vi "ALP2 P.vi"() -> ()   [LabVIEW 2016]
doc: "This VI starts running and asks if it want to adquire data or exit. If the user choose to adquired data the user is allowed to make dynamic changes to the resulting graph so it can best fit the data, also it allows the user to save the data and the folder is already named with the date and time the data was saved. It allows to make a header to the data which is included in the file.\n\nAlexis Lopez\nP350\nCSUSB Physics"
uses:
  typedefs/measurement parameters.ctl
  typedefs/ferro response parameter cluster.ctl
panel:
  in  "date format (0) 2":enum16{"short", "long", "abbreviated"}(ring)
  in  "Stop":bool
  in  "File Header":string="This run was taken on the XXX sample under the following conditions: Temp=..., etc. ...\n\nFormat:\ntime    voltage    fit voltage    fit parameters\n\n<data below>\n\n"
  out "Data to Save":dbl[][](array[numeric])
  in  "Restart":bool
  in  "Save Data":bool
  in  "Fitting Parameters":T1={"amplitude a (V)"=5.0, "time const a (uS)"=15.0, "amplitude b (V)"=10.0, "time const b (uS)"=150.0} {"time const b (uS)" scale=0.0..200.0; "amplitude b (V)" scale=0.0..50.0; "time const a (uS)" scale=0.0..200.0; "amplitude a (V)" scale=0.0..50.0}
  out "Analysis Graph":cluster{"time array (s)":dbl[], dbl[]}[](graph)
  out "Acquisition Graph":T2(graph)
  out "count":i32=100
  in  "Meas Params":T3={"time step (uS)"=1.0, "N meas"=1000, "N meas reps"=100} caption="Measurement Parameters"
  in  "Start":bool
  # "Simulated FerroElectric Experiment"
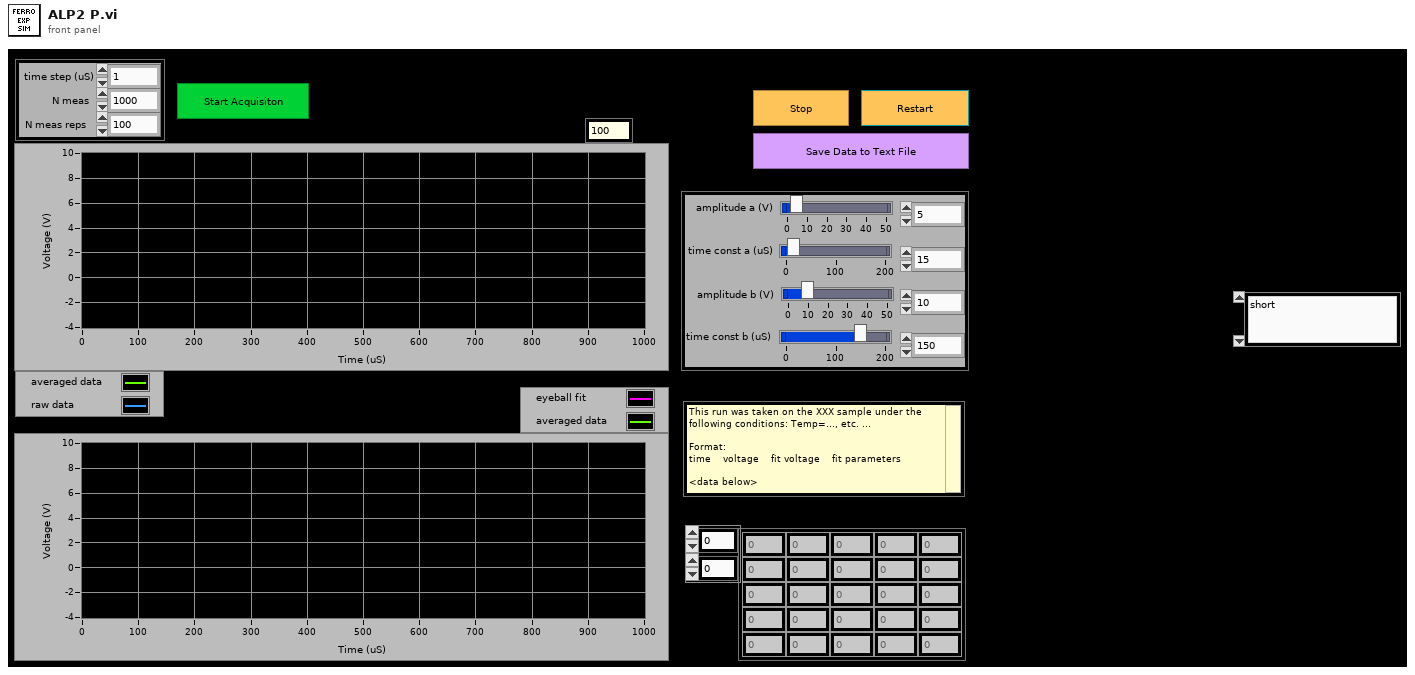
[diagram p1: front panel]
types:
  T1 = typedef "ferro response parameter cluster.ctl" = cluster{"amplitude a (V)":dbl, "time const a (uS)":dbl, "amplitude b (V)":dbl, "time const b (uS)":dbl}
  T2 = cluster{"time array (s)":dbl[], "voltage array (V)":dbl[]}[]
  T3 = typedef "measurement parameters.ctl" = cluster{"time step (uS)":dbl, "N meas":i32, "N meas reps":i32}
  T4 = cluster{"time array (uS)":dbl[], "voltage array (V)":dbl[]}
  T5 = cluster{"time array (uS)":dbl[], "voltage array (V)":dbl[]}[]
  T6 = cluster{"time array out (uS)":dbl[], "voltage array out (V)":dbl[]}
  T7 = cluster{"time array out (uS)":dbl[], "voltage array out (V)":dbl[]}[]
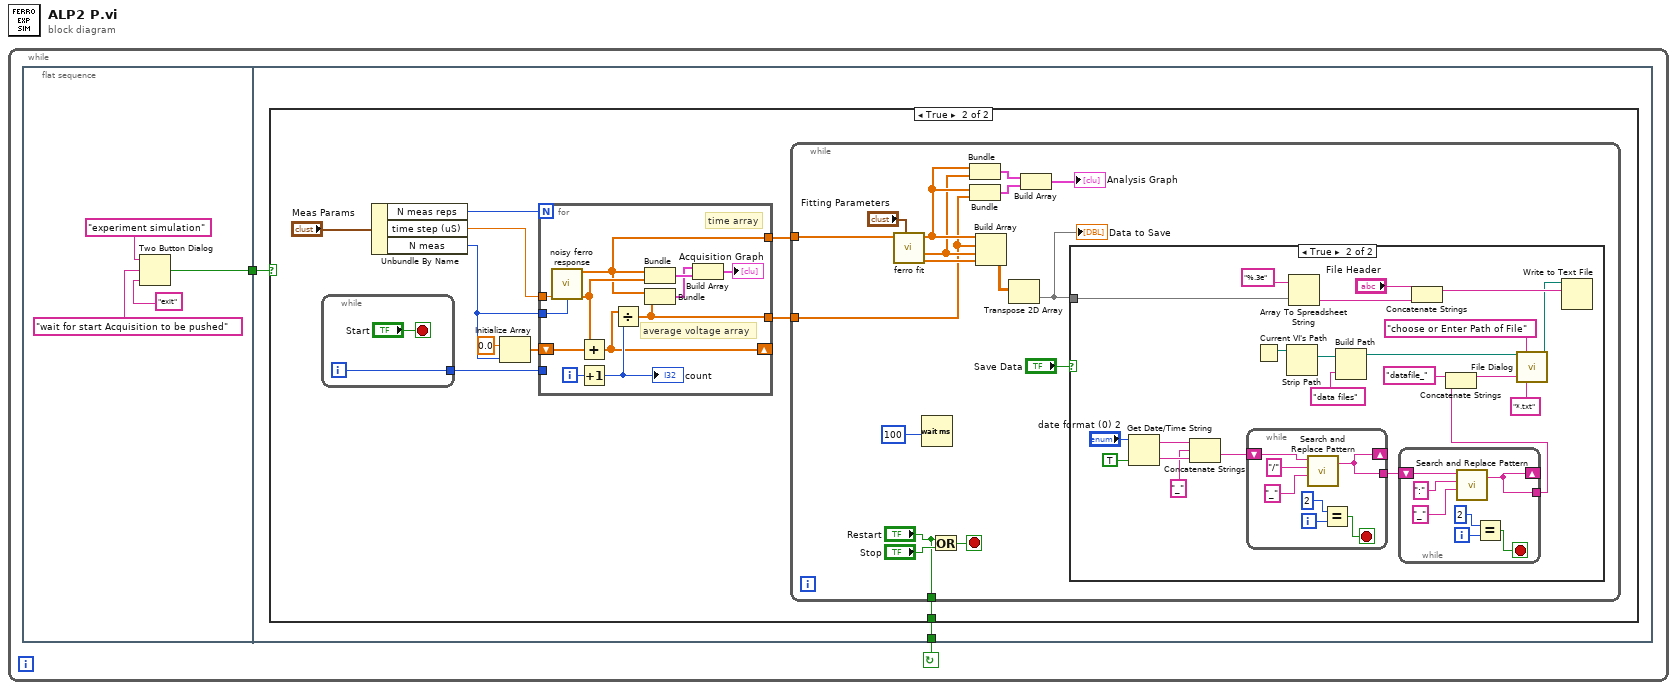
[diagram p0: block diagram]
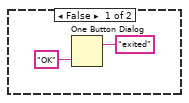
[diagram p2: hidden frame]
diagram:
  n1 = while {
    stop <- w1 continue-if-true
    n2 = flat-sequence {
      tunnel: [w3] -> w2
      tunnel: w2 -> [w8]
      tunnel: [w7] -> w1
      frame #0 {
        n3 = Two Button Dialog(message="experiment simulation", 1:"exit", 2:"wait for start Acquisition to be pushed") -> (T button?=w3:bool)
      }
      frame #1 {
        n4 = case shown="True" w8 {
          tunnel: [_ w11] -> w7
          frame False {
            n5 = One Button Dialog(message="exited", button name ("OK")="OK") -> ()  [unwired: 1 out]
          }
          frame True {
            n6 = while {
              tunnel: [w21] -> w12
              i -> [w21]
              stop <- "Start" stop-if-true
            }
            n7 = Unbundle By Name("Meas Params") -> ("N meas reps"=w15:i32, "time step (uS)"=w19:dbl, "N meas"=w16:i32)
            n8 = Initialize Array(0.0 ("element"), w16) -> (w18:dbl[])
            n9 = for {
              N: w15 -> [_]
              tunnel: w19 -> [w86]
              tunnel: w16 -> [w85]
              shift-right: [w79] -> _
              shift-left: w18 -> [w80]
              tunnel: [w76] -> w14
              tunnel: [w75] -> w13
              tunnel: w12 -> [_]
              i -> [w84]
              # "average voltage array"
              # "time array"
              n10 = call "noisy ferro response.vi"("time step (uS)"=w86, "N meas"=w85) -> ("time array (uS)"=w76:dbl[], "voltage array (V)"=w81:dbl[])  [unwired: 12 in]
              n11 = Add(x=w81, y=w80) -> (x+y=w79:dbl[])
              n12 = Increment(x=w84) -> (x+1=w83:i32)
              "count" <- w83
              n13 = Divide(x=w79, y=w83) -> (x/y=w75:dbl[])
              n14 = Bundle("time array (uS)"=w76, "voltage array (V)"=w81) -> (w78:T4)  [unwired: 1 in]
              n15 = Bundle("time array (uS)"=w76, w75) -> (w77:cluster{"time array (uS)":dbl[], dbl[]})  [unwired: 1 in]
              n16 = Build Array(w77, w78) -> (→"Acquisition Graph":T5)
            }
            n17 = while {
              tunnel: w14 -> [w37]
              tunnel: w13 -> [w28]
              tunnel: ["Restart"] -> w11
              stop <- w24 stop-if-true
              n18 = call "ferro fit.vi"("ferro response parameters"="Fitting Parameters", "time array in (uS)"=w37) -> ("parameters array out"=w31:dbl[], "voltage array out (V)"=w29:dbl[], "time array out (uS)"=w30:dbl[])  [unwired: 7 in]
              n19 = Wait (ms)(milliseconds to wait=u32 100 ("millisecond timer value")) -> ()  [unwired: 1 out]
              n20 = Or(x="Restart", y="Stop") -> (x .or. y?=w24:bool)
              n21 = Bundle("time array out (uS)"=w30, "voltage array out (V)"=w29) -> (w34:T6)  [unwired: 1 in]
              n22 = Bundle("time array out (uS)"=w30, w28) -> (w33:cluster{"time array out (uS)":dbl[], dbl[]})  [unwired: 1 in]
              n23 = Build Array(w30, w28, w29, w31) -> (w35:dbl[][])
              n24 = Transpose 2D Array(2D array=w35) -> (transposed array=w26:dbl[][])
              "Data to Save" <- w26
              n25 = Build Array(w34, w33) -> (→"Analysis Graph":T7)
              n26 = case shown="True" "Save Data" {
                tunnel: w26 -> [_ w60]
                frame False {
                }
                frame True {
                  n27 = Get Date/Time String(date format (0)="date format (0) 2", want seconds? (F)=TRUE) -> (date string=w41:string, time string=w46:string)  [unwired: 1 in]
                  n28 = Concatenate Strings(w41, "_", w46) -> (w44:string)
                  n29 = while {
                    shift-right: [w73] -> _
                    shift-left: w44 -> [w74]
                    tunnel: [w73] -> w45
                    i -> [w72]
                    stop <- w70 stop-if-true
                    n30 = call <vilib>:"Search and Replace Pattern.vi"("string"=w74, "regular expression (\"\")"="/", "replace string (\"\")"="_") -> ("result string"=w73:string)  [unwired: 2 in, 1 out]
                    n31 = Equal?(x=2, y=w72) -> (x = y?=w70:bool)
                  }
                  n32 = Current VI's Path() -> (path=w55:path)
                  n33 = Strip Path(path=w55) -> (stripped path=w49:path)  [unwired: 1 out]
                  n34 = Array To Spreadsheet String(array=w60, 3:"%.3e") -> (spreadsheet string=w57:string)  [unwired: 1 in]
                  n35 = Build Path(base path=w49, name or relative path="data files") -> (appended path=w53:path)
                  n36 = while {
                    shift-right: [w66] -> _
                    shift-left: w45 -> [w67]
                    tunnel: [w66] -> w39
                    i -> [w63]
                    stop <- w64 stop-if-true
                    n37 = call <vilib>:"Search and Replace Pattern.vi"("string"=w67, "regular expression (\"\")"=":", "replace string (\"\")"="_") -> ("result string"=w66:string)  [unwired: 2 in, 1 out]
                    n38 = Equal?(x=2, y=w63) -> (x = y?=w64:bool)
                  }
                  n39 = Concatenate Strings("File Header", w57) -> (w58:string)
                  n40 = Concatenate Strings("datafile_", w39) -> (w42:string)
                  n41 = call "File Dialog"("start path"=w53, "prompt"="choose or Enter Path of File", "default name"=w42, "pattern (all files)"="*.txt") -> ("selected path"=w50:path)  [unwired: 8 in, 3 out]
                  n42 = Write to Text File(file (use dialog)=w50, text=w58) -> ()  [unwired: 2 in, 3 out]
                }
              }
            }
          }
        }
      }
    }
  }
